vi "SaveData.vi"(0 "TDMS Logging in":refnum<class "TDMS Logging.lvclass">, 1 "Path Control":path, 2 "Signal":dbl[](graph), 3 "error in (no error)":errorcluster) -> (7 "TDMS Logging out":refnum<class "TDMS Logging.lvclass">, 10 "error out":errorcluster)   [LabVIEW 2020, in "TDMS Logging.lvlib" / "TDMS Logging.lvclass"]
uses:
  TDMS Logging.lvclass
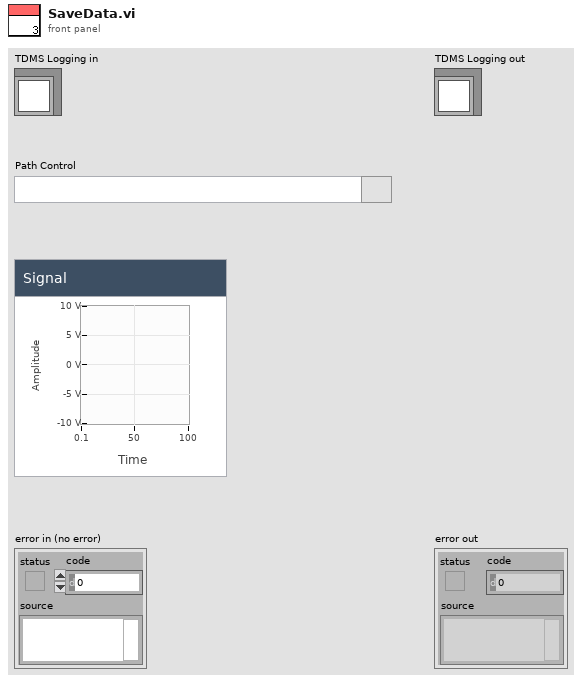
[diagram p1: front panel]
types:
  T1 = enum16{"open", "open or create", "create or replace", "create", "open (read-only)"}
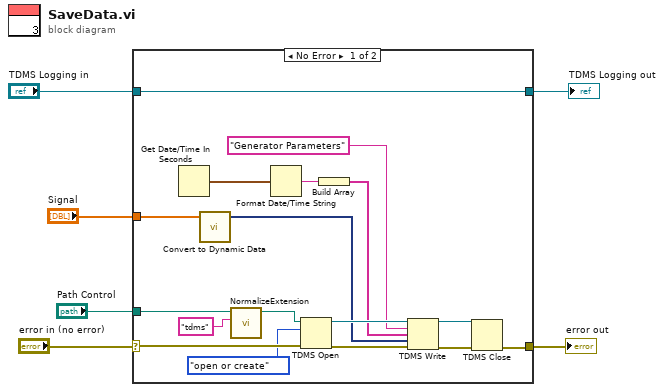
[diagram p0: block diagram]
diagram:
  n1 = case shown="No Error" "error in (no error)" {
    selector: "error in (no error)" -> [w19 w24]
    tunnel: "TDMS Logging in" -> [w23 w25]
    tunnel: [w23 w25] -> w1
    tunnel: [w7 w24] -> w2
    tunnel: "Path Control" -> [w22 _]
    tunnel: "Signal" -> [w20 _]
    frame No Error {
      n2 = Get Date/Time In Seconds() -> (seconds since 1Jan1904=w13:timestamp)
      n3 = call "Convert to Dynamic Data"("Array"=w20) -> ("Dynamic Data Type"=w10:dynamicdata)  [unwired: 3 in]
      n4 = call "NormalizeExtension.vi"("Extension"="tdms", "Path in"=w22) -> ("Path out"=w18:path)  [unwired: 9 in]
      n5 = Format Date/Time String(seconds (now)=w13) -> (date/time string=w12:string)  [unwired: 2 in]
      n6 = TDMS Open(8:w19, 10:T1."open or create" ("operation (0:open)"), 11:w18) -> (0:w15:errorcluster, 3:w16:refnum<k34>)  [unwired: 4 in]
      n7 = Build Array(w12) -> (w11:string[])
      n8 = TDMS Write(0:w16, 5:"Generator Parameters" ("group name in (Untitled)"), 7:w11, 9:w10, 11:w15) -> (4:w8:refnum<k34>, 15:w9:errorcluster)  [unwired: 1 in, 2 out]
      n9 = TDMS Close(8:w9, 11:w8) -> (0:w7:errorcluster)  [unwired: 1 out]
    }
    frame Error {
    }
  }
  "error out" <- w2
  "TDMS Logging out" <- w1
